vi "Weather Parse Test.vi"() -> ()   [LabVIEW 2020, in "CDM-Config.lvlib"] (continued)
\"NationalWeatherService\": [\n                        \"SCY\"\n                    ]\n                }\n            }\n        },\n        {\n            \"id\": \"https://api.weather.gov/alerts/urn:oid:2.49.0.1.840.0.85cfcb06bd0c86092fff4359af75aac0fabec681.004.1\",\n            \"type\": \"Feature\",\n            \"geometry\": null,\n            \"properties\": {\n                \"@id\": \"https://api.weather.gov/alerts/urn:oid:2.49.0.1.840.0.85cfcb06bd0c86092fff4359af75aac0fabec681.004.1\",\n                \"@type\": \"wx:Alert\",\n                \"id\": \"urn:oid:2.49.0.1.840.0.85cfcb06bd0c86092fff4359af75aac0fabec681.004.1\",\n                \"areaDesc\": \"Coastal waters from Cape Mendocino to Pt. Arena CA out 10 nm\",\n                \"geocode\": {\n                    \"SAME\": [\n                        \"057455\"\n                    ],\n                    \"UGC\": [\n                        \"PZZ455\"\n                    ]\n                },\n                \"affectedZones\": [\n                    \"https://api.weather.gov/zones/forecast/PZZ455\"\n                ],\n                \"references\": [\n                    {\n                        \"@id\": \"https://api.weather.gov/alerts/urn:oid:2.49.0.1.840.0.60f47e7d527764f0ce222d0fcb908b2519fae517.003.1\",\n                        \"identifier\": \"urn:oid:2.49.0.1.840.0.60f47e7d527764f0ce222d0fcb908b2519fae517.003.1\",\n                        \"sender\": \"w-nws.webmaster@noaa.gov\",\n                        \"sent\": \"2025-12-03T03:17:00-08:00\"\n                    }\n                ],\n                \"sent\": \"2025-12-03T07:39:00-08:00\",\n                \"effective\": \"2025-12-03T07:39:00-08:00\",\n                \"onset\": \"2025-12-03T07:39:00-08:00\",\n                \"expires\": \"2025-12-03T10:00:00-08:00\",\n                \"ends\": \"2025-12-03T10:00:00-08:00\",\n                \"status\": \"Actual\",\n                \"messageType\": \"Update\",\n                \"category\": \"Met\",\n                \"severity\": \"Minor\",\n                \"certainty\": \"Likely\",\n                \"urgency\": \"Expected\",\n                \"event\": \"Small Craft Advisory\",\n                \"sender\": \"w-nws.webmaster@noaa.gov\",\n                \"senderName\": \"NWS Eureka CA\",\n                \"headline\": \"Small Craft Advisory issued December 3 at 7:39AM PST until December 3 at 10:00AM PST by NWS Eureka CA\",\n                \"description\": \"* WHAT...North winds 10 to 20 kt with gusts up to 25 kt and seas\\n8 to 10 feet.\\n\\n* WHERE...Cape Mendocino to Pt Arena out 10 nm.\\n\\n* WHEN...Until 10 AM PST this morning.\\n\\n* IMPACTS...Conditions will be hazardous to small craft.\",\n                \"instruction\": \"Inexperienced mariners, especially those operating smaller\\nvessels, should avoid navigating in hazardous conditions.\",\n                \"response\": \"Avoid\",\n                \"parameters\": {\n                    \"AWIPSidentifier\": [\n                        \"MWWEKA\"\n                    ],\n                    \"WMOidentifier\": [\n                        \"WHUS76 KEKA 031539\"\n                    ],\n                    \"NWSheadline\": [\n                        \"SMALL CRAFT ADVISORY REMAINS IN EFFECT UNTIL 10 AM PST THIS MORNING\"\n                    ],\n                    \"BLOCKCHANNEL\": [\n                        \"EAS\",\n                        \"NWEM\",\n                        \"CMAS\"\n                    ],\n                    \"VTEC\": [\n                        \"/O.CON.KEKA.SC.Y.0131.000000T0000Z-251203T1800Z/\"\n                    ],\n                    \"eventEndingTime\": [\n                        \"2025-12-03T10:00:00-08:00\"\n                    ],\n                    \"expiredReferences\": [\n                        \"w-nws.webmaster@noaa.gov,urn:oid:2.49.0.1.840.0.abe195d0561fd25b031b5bfec9df0b944a5ace40.003.1,2025-12-02T21:50:00-08:00 w-nws.webmaster@noaa.gov,urn:oid:2.49.0.1.840.0.e32ecb5cf39de3c0d1e2da73c56319d7880d5ad3.004.1,2025-12-02T15:45:00-08:00 w-nws.webmaster@noaa.gov,urn:oid:2.49.0.1.840.0.e0b91c1e8c9c801e386b75444bbd2a0bbc5299eb.004.1,2025-12-02T14:39:00-08:00 w-nws.webmaster@noaa.gov,urn:oid:2.49.0.1.840.0.0a5dc3462cdc1726ad314e876783ee5bf7071762.004.1,2025-12-02T09:55:00-08:00 w-nws.webmaster@noaa.gov,urn:oid:2.49.0.1.840.0.01de2552a96f0b556f81f7a24cea9bae9b7d39b8.003.1,2025-12-02T03:48:00-08:00 w-nws.webmaster@noaa.gov,urn:oid:2.49.0.1.840.0.ca2f9b9bc4efc4c7ec6c14c74d7b35cc28fee802.003.1,2025-12-01T20:59:00-08:00 w-nws.webmaster@noaa.gov,urn:oid:2.49.0.1.840.0.341d2d3541a24810a337eb1f7ebd4af858289c9a.003.1,2025-12-01T14:59:00-08:00 w-nws.webmaster@noaa.gov,urn:oid:2.49.0.1.840.0.e0da5ffb117eb3eb07d4855bb3809c65d8bd08ee.001.1,2025-11-30T22:46:00-08:00 w-nws.webmaster@noaa.gov,urn:oid:2.49.0.1.840.0.3141b440711a7dab2caf67b4d892f368eedce3a1.001.1,2025-11-30T15:10:00-08:00 w-nws.webmaster@noaa.gov,urn:oid:2.49.0.1.840.0.61c600a3fee31e0c5b3344407f02fbb11b4030f7.003.1,2025-11-30T11:25:00-08:00 w-nws.webmaster@noaa.gov,urn:oid:2.49.0.1.840.0.475fbd03966c809e753c380c88b8f5a7913fc370.001.1,2025-11-30T02:23:00-08:00 w-nws.webmaster@noaa.gov,urn:oid:2.49.0.1.840.0.456ac22e39df6d72b640469b5ee3cd6819367cee.001.1,2025-11-29T22:41:00-08:00 w-nws.webmaster@noaa.gov,urn:oid:2.49.0.1.840.0.3f2569b420bbe6dab1f5676473753e2d387027f5.001.1,2025-11-29T15:01:00-08:00 w-nws.webmaster@noaa.gov,urn:oid:2.49.0.1.840.0.558b96257a3d492dbe31195be5d89212c36df85e.003.1,2025-11-29T10:51:00-08:00 w-nws.webmaster@noaa.gov,urn:oid:2.49.0.1.840.0.96be26edb9a6c9dcbf7df831b0453d5650027364.001.1,2025-11-29T02:25:00-08:00 w-nws.webmaster@noaa.gov,urn:oid:2.49.0.1.840.0.c3b1f937b5abbc5ea56d2724b02e758aa1c01179.002.1,2025-11-28T22:31:00-08:00 w-nws.webmaster@noaa.gov,urn:oid:2.49.0.1.840.0.e3db8e512cec14c9022bfe9f2c10ba787d2e6b8d.001.1,2025-11-28T11:48:00-08:00\"\n                    ]\n                },\n                \"scope\": \"Public\",\n                \"code\": \"IPAWSv1.0\",\n                \"language\": \"en-US\",\n                \"web\": \"http://www.weather.gov\",\n                \"eventCode\": {\n                    \"SAME\": [\n                        \"NWS\"\n                    ],\n                    \"NationalWeatherService\": [\n                        \"SCY\"\n                    ]\n                }\n            }\n        },\n        {\n            \"id\": \"https://api.weather.gov/alerts/urn:oid:2.49.0.1.840.0.220f0a3be3b6cd2f2d64124491430aaf409f9b6f.001.1\",\n            \"type\": \"Feature\",\n            \"geometry\": null,\n            \"properties\": {\n                \"@id\": \"https://api.weather.gov/alerts/urn:oid:2.49.0.1.840.0.220f0a3be3b6cd2f2d64124491430aaf409f9b6f.001.1\",\n                \"@type\": \"wx:Alert\",\n                \"id\": \"urn:oid:2.49.0.1.840.0.220f0a3be3b6cd2f2d64124491430aaf409f9b6f.001.1\",\n                \"areaDesc\": \"Western Chippewa; Central Chippewa\",\n                \"geocode\": {\n                    \"SAME\": [\n                        \"026033\"\n                    ],\n                    \"UGC\": [\n                        \"MIZ086\",\n                        \"MIZ087\"\n                    ]\n                },\n                \"affectedZones\": [\n                    \"https://api.weather.gov/zones/forecast/MIZ086\",\n                    \"https://api.weather.gov/zones/forecast/MIZ087\"\n                ],\n                \"references\": [\n                    {\n                        \"@id\": \"https://api.weather.gov/alerts/urn:oid:2.49.0.1.840.0.68f3b48d66caf3405fc5bfbb1a371148b61f2b0f.001.1\",\n                        \"identifier\": \"urn:oid:2.49.0.1.840.0.68f3b48d66caf3405fc5bfbb1a371148b61f2b0f.001.1\",\n                        \"sender\": \"w-nws.webmaster@noaa.gov\",\n                        \"sent\": \"2025-12-03T02:53:00-05:00\"\n                    }\n                ],\n                \"sent\": \"2025-12-03T10:36:00-05:00\",\n                \"effective\": \"2025-12-03T10:36:00-05:00\",\n                \"onset\": \"2025-12-03T13:00:00-05:00\",\n                \"expires\": \"2025-12-03T22:45:00-05:00\",\n                \"ends\": \"2025-12-04T13:00:00-05:00\",\n                \"status\": \"Actual\",\n                \"messageType\": \"Update\",\n                \"category\": \"Met\",\n                \"severity\": \"Severe\",\n                \"certainty\": \"Likely\",\n                \"urgency\": \"Expected\",\n                \"event\": \"Winter Storm Warning\",\n                \"sender\": \"w-nws.webmaster@noaa.gov\",\n                \"senderName\": \"NWS Gaylord MI\",\n                \"headline\": \"Winter Storm Warning issued December 3 at 10:36AM EST until December 4 at 1:00PM EST by NWS Gaylord MI\",\n                \"description\": \"* WHAT...Heavy snow expected. Total snow accumulations between 6 and\\n12 inches, locally higher amounts possible. Winds gusting between\\n25 and 30 mph will result in blowing snow at times.\\n\\n* WHERE...Central Chippewa and Western Chippewa Counties.\\n\\n* WHEN...Until 1 PM EST Thursday.\\n\\n* IMPACTS...Visibilities may drop below 1/4 mile due to falling and\\nblowing snow. Travel could be very difficult. The hazardous\\nconditions will impact the Thursday morning commute.\",\n                \"instruction\": \"If you must travel, keep an extra flashlight, food, and water in\\nyour vehicle in case of an emergency.\\n\\nIf travel is absolutely necessary, drive with extreme caution and be\\nprepared for sudden changes in visibility. Leave plenty of room\\nbetween you and the motorist ahead of you, and allow extra time to\\nreach your destination. Avoid sudden braking or acceleration, and be\\nespecially cautious on hills or when making turns. Make sure your\\ncar is winterized and in good working order.\",\n                \"response\": \"Prepare\",\n                \"parameters\": {\n                    \"AWIPSidentifier\": [\n                        \"WSWAPX\"\n                    ],\n                    \"WMOidentifier\": [\n                        \"WWUS43 KAPX 031536\"\n                    ],\n                    \"NWSheadline\": [\n                        \"WINTER STORM WARNING REMAINS IN EFFECT UNTIL 1 PM EST THURSDAY\"\n                    ],\n                    \"BLOCKCHANNEL\": [\n                        \"EAS\",\n                        \"NWEM\",\n                        \"CMAS\"\n                    ],\n                    \"EAS-ORG\": [\n                        \"WXR\"\n                    ],\n                    \"VTEC\": [\n                        \"/O.CON.KAPX.WS.W.0014.251203T1800Z-251204T1800Z/\"\n                    ],\n                    \"eventEndingTime\": [\n                        \"2025-12-04T13:00:00-05:00\"\n                    ]\n                },\n                \"scope\": \"Public\",\n                \"code\": \"IPAWSv1.0\",\n                \"language\": \"en-US\",\n                \"web\": \"http://www.weather.gov\",\n                \"eventCode\": {\n                    \"SAME\": [\n                        \"WSW\"\n                    ],\n                    \"NationalWeatherService\": [\n                        \"WSW\"\n                    ]\n                }\n            }\n        },\n        {\n            \"id\": \"https://api.weather.gov/alerts/urn:oid:2.49.0.1.840.0.70532f7794760aa59fb14677883cbb330aad0f90.001.1\",\n            \"type\": \"Feature\",\n            \"geometry\": null,\n            \"properties\": {\n                \"@id\": \"https://api.weather.gov/alerts/urn:oid:2.49.0.1.840.0.70532f7794760aa59fb14677883cbb330aad0f90.001.1\",\n                \"@type\": \"wx:Alert\",\n                \"id\": \"urn:oid:2.49.0.1.840.0.70532f7794760aa59fb14677883cbb330aad0f90.001.1\",\n                \"areaDesc\": \"New Buffalo MI to St Joseph MI; Michigan City IN to New Buffalo MI\",\n                \"geocode\": {\n                    \"SAME\": [\n                        \"092043\",\n                        \"092046\"\n                    ],\n                    \"UGC\": [\n                        \"LMZ043\",\n                        \"LMZ046\"\n                    ]\n                },\n                \"affectedZones\": [\n                    \"https://api.weather.gov/zones/forecast/LMZ043\",\n                    \"https://api.weather.gov/zones/forecast/LMZ046\"\n                ],\n                \"references\": [\n                    {\n                        \"@id\": \"https://api.weather.gov/alerts/urn:oid:2.49.0.1.840.0.875506e3e040bbcc4b2fc71b1eece95556c3b51a.001.1\",\n                        \"identifier\": \"urn:oid:2.49.0.1.840.0.875506e3e040bbcc4b2fc71b1eece95556c3b51a.001.1\",\n                        \"sender\": \"w-nws.webmaster@noaa.gov\",\n                        \"sent\": \"2025-12-03T04:19:00-05:00\"\n                    }\n                ],\n                \"sent\": \"2025-12-03T10:28:00-05:00\",\n                \"effective\": \"2025-12-03T10:28:00-05:00\",\n                \"onset\": \"2025-12-03T10:28:00-05:00\",\n                \"expires\": \"2025-12-03T18:30:00-05:00\",\n                \"ends\": \"2025-12-04T19:00:00-05:00\",\n                \"status\": \"Actual\",\n                \"messageType\": \"Update\",\n                \"category\": \"Met\",\n                \"severity\": \"Minor\",\n                \"certainty\": \"Likely\",\n                \"urgency\": \"Expected\",\n                \"event\": \"Small Craft Advisory\",\n                \"sender\": \"w-nws.webmaster@noaa.gov\",\n                \"senderName\": \"NWS Northern Indiana\",\n                \"headline\": \"Small Craft Advisory issued December 3 at 10:28AM EST until December 4 at 7:00PM EST by NWS Northern Indiana\",\n                \"description\": \"* WHAT...Southwest 15 to 25 knots becoming northwest with gusts\\nup to 25 to 30 knots and waves 6 to 9 feet.\\n\\n* WHERE...Michigan City IN to St Joseph MI.\\n\\n* WHEN...Until 7 PM EST Thursday.\\n\\n* IMPACTS...Conditions will be hazardous to small craft.\",\n                \"instruction\": \"Inexperienced mariners, especially those operating smaller\\nvessels, should avoid navigating in hazardous conditions.\",\n                \"response\": \"Avoid\",\n                \"parameters\": {\n                    \"AWIPSidentifier\": [\n                        \"MWWIWX\"\n                    ],\n                    \"WMOidentifier\": [\n                        \"WHUS73 KIWX 031528\"\n                    ],\n                    \"NWSheadline\": [\n                        \"SMALL CRAFT ADVISORY REMAINS IN EFFECT UNTIL 7 PM EST THURSDAY\"\n                    ],\n                    \"BLOCKCHANNEL\": [\n                        \"EAS\",\n                        \"NWEM\",\n                        \"CMAS\"\n                    ],\n                    \"VTEC\": [\n                        \"/O.CON.KIWX.SC.Y.0073.000000T0000Z-251205T0000Z/\"\n                    ],\n                    \"eventEndingTime\": [\n                        \"2025-12-04T19:00:00-05:00\"\n                    ],\n                    \"expiredReferences\": [\n                        \"w-nws.webmaster@noaa.gov,urn:oid:2.49.0.1.840.0.225142cd75165574bdad700dfb60a5d5354b40a4.001.1,2025-12-02T21:13:00-05:00 w-nws.webmaster@noaa.gov,urn:oid:2.49.0.1.840.0.a0e704ec5a442f14cfca1d10613311a0e02b15c6.001.1,2025-12-02T15:47:00-05:00 w-nws.webmaster@noaa.gov,urn:oid:2.49.0.1.840.0.6b2791b857a86681ce998af8adb83a08b01f25a5.001.1,2025-12-02T11:04:00-05:00 w-nws.webmaster@noaa.gov,urn:oid:2.49.0.1.840.0.a57567c3b2042ce4a02e8b09eda0f6c7e7ccc8d7.001.1,2025-12-02T03:51:00-05:00\"\n                    ]\n                },\n                \"scope\": \"Public\",\n                \"code\": \"IPAWSv1.0\",\n                \"language\": \"en-US\",\n                \"web\": \"http://www.weather.gov\",\n                \"eventCode\": {\n                    \"SAME\": [\n                        \"NWS\"\n                    ],\n                    \"NationalWeatherService\": [\n                        \"SCY\"\n                    ]\n                }\n            }\n        },\n        {\n            \"id\": \"https://api.weather.gov/alerts/urn:oid:2.49.0.1.840.0.296069c17a90f6e5215450afb7029362483104e1.002.1\",\n            \"type\": \"Feature\",\n            \"geometry\": null,\n            \"properties\": {\n                \"@id\": \"https://api.weather.gov/alerts/urn:oid:2.49.0.1.840.0.296069c17a90f6e5215450afb7029362483104e1.002.1\",\n                \"@type\": \"wx:Alert\",\n                \"id\": \"urn:oid:2.49.0.1.840.0.296069c17a90f6e5215450afb7029362483104e1.002.1\",\n                \"areaDesc\": \"Northern Sangre de Cristo Mountains Between 8500 And 11000 Ft; Northern Sangre de Cristo Mountains above 11000 Ft; Southern Sangre De Cristo Mountains Between 7500 and 11000 Ft; Southern Sangre De Cristo Mountains Above 11000 Ft\",\n                \"geocode\": {\n                    \"SAME\": [\n                        \"008003\",\n                        \"008015\",\n                        \"008023\",\n                        \"008027\",\n                        \"008043\",\n                        \"008055\",\n                        \"008109\",\n                        \"008071\"\n                    ],\n                    \"UGC\": [\n                        \"COZ072\",\n                        \"COZ073\",\n                        \"COZ074\",\n                        \"COZ075\"\n                    ]\n                },\n                \"affectedZones\": [\n                    \"https://api.weather.gov/zones/forecast/COZ072\",\n                    \"https://api.weather.gov/zones/forecast/COZ073\",\n                    \"https://api.weather.gov/zones/forecast/COZ074\",\n                    \"https://api.weather.gov/zones/forecast/COZ075\"\n                ],\n                \"references\": [\n                    {\n                        \"@id\": \"https://api.weather.gov/alerts/urn:oid:2.49.0.1.840.0.f1520a771888f2286c7e9f041b0899cca2ffbe10.001.1\",\n                        \"identifier\": \"urn:oid:2.49.0.1.840.0.f1520a771888f2286c7e9f041b0899cca2ffbe10.001.1\",\n                        \"sender\": \"w-nws.webmaster@noaa.gov\",\n                        \"sent\": \"2025-12-03T00:40:00-07:00\"\n                    },\n                    {\n                        \"@id\": \"https://api.weather.gov/alerts/urn:oid:2.49.0.1.840.0.3e97ab4a6a3c23a3a20405d82b018ef9927db31d.002.1\",\n                        \"identifier\": \"urn:oid:2.49.0.1.840.0.3e97ab4a6a3c23a3a20405d82b018ef9927db31d.002.1\",\n                        \"sender\": \"w-nws.webmaster@noaa.gov\",\n                        \"sent\": \"2025-12-03T00:46:00-07:00\"\n                    },\n                    {\n                        \"@id\": \"https://api.weather.gov/alerts/urn:oid:2.49.0.1.840.0.b7b2384d0cd65fff536137c85933eace889e9254.001.1\",\n                        \"identifier\": \"urn:oid:2.49.0.1.840.0.b7b2384d0cd65fff536137c85933eace889e9254.001.1\",\n                        \"sender\": \"w-nws.webmaster@noaa.gov\",\n                        \"sent\": \"2025-12-03T00:53:00-07:00\"\n                    },\n                    {\n                        \"@id\": \"https://api.weather.gov/alerts/urn:oid:2.49.0.1.840.0.5bb2b589973a618ffa88ed552c21d1806fce1897.001.1\",\n                        \"identifier\": \"urn:oid:2.49.0.1.840.0.5bb2b589973a618ffa88ed552c21d1806fce1897.001.1\",\n                        \"sender\": \"w-nws.webmaster@noaa.gov\",\n                        \"sent\": \"2025-12-03T02:10:00-07:00\"\n                    }\n                ],\n                \"sent\": \"2025-12-03T08:17:00-07:00\",\n                \"effective\": \"2025-12-03T08:17:00-07:00\",\n                \"onset\": \"2025-12-03T08:17:00-07:00\",\n                \"expires\": \"2025-12-03T16:30:00-07:00\",\n                \"ends\": \"2025-12-04T02:00:00-07:00\",\n                \"status\": \"Actual\",\n                \"messageType\": \"Update\",\n                \"category\": \"Met\",\n                \"severity\": \"Severe\",\n                \"certainty\": \"Likely\",\n                \"urgency\": \"Expected\",\n                \"event\": \"Winter Storm Warning\",\n                \"sender\": \"w-nws.webmaster@noaa.gov\",\n                \"senderName\": \"NWS Pueblo CO\",\n                \"headline\": \"Winter Storm Warning issued December 3 at 8:17AM MST until December 4 at 2:00AM MST by NWS Pueblo CO\",\n                \"description\": \"* WHAT...Heavy snow expected. Total snow accumulations between 8 to\\n20 inches.\\n\\n* WHERE...Sangre de Cristo Mountains.\\n\\n* WHEN...Until 2 AM MST Thursday.\\n\\n* IMPACTS...Travel could be very difficult to impossible. The\\nhazardous conditions could impact the Wednesday evening commute.\",\n                \"instruction\": \"If you must travel, keep an extra flashlight, food, and water in\\nyour vehicle in case of an emergency. The latest road conditions for\\nthe state you are calling from can be obtained by calling 5 1 1.\\n\\nPersons should consider delaying all travel. Motorists should use\\nextreme caution if travel is absolutely necessary.\",\n                \"response\": \"Prepare\",\n                \"parameters\": {\n                    \"AWIPSidentifier\": [\n                        \"WSWPUB\"\n                    ],\n                    \"WMOidentifier\": [\n                        \"WWUS45 KPUB 031517\"\n                    ],\n                    \"NWSheadline\": [\n                        \"WINTER STORM WARNING REMAINS IN EFFECT UNTIL 2 AM MST THURSDAY\"\n                    ],\n                    \"BLOCKCHANNEL\": [\n                        \"EAS\",\n                        \"NWEM\",\n                        \"CMAS\"\n                    ],\n                    \"EAS-ORG\": [\n                        \"WXR\"\n                    ],\n                    \"VTEC\": [\n                        \"/O.CON.KPUB.WS.W.0011.000000T0000Z-251204T0900Z/\"\n                    ],\n                    \"eventEndingTime\": [\n                        \"2025-12-04T02:00:00-07:00\"\n                    ],\n                    \"expiredReferences\": [\n                        \"w-nws.webmaster@noaa.gov,urn:oid:2.49.0.1.840.0.1683fac8dbbcced155b8c3ee102b504a61d03b48.001.1,2025-12-02T21:22:00-07:00 w-nws.webmaster@noaa.gov,urn:oid:2.49.0.1.840.0.3af7c19979dcb0fd957b60f169e1bc971c265b37.001.2,2025-12-02T14:07:00-07:00\"\n                    ]\n                },\n                \"scope\": \"Public\",\n                \"code\": \"IPAWSv1.0\",\n                \"language\": \"en-US\",\n                \"web\": \"http://www.weather.gov\",\n                \"eventCode\": {\n                    \"SAME\": [\n                        \"WSW\"\n                    ],\n                    \"NationalWeatherService\": [\n                        \"WSW\"\n                    ]\n                }\n            }\n        },\n        {\n            \"id\": \"https://api.weather.gov/alerts/urn:oid:2.49.0.1.840.0.296069c17a90f6e5215450afb7029362483104e1.001.2\",\n            \"type\": \"Feature\",\n            \"geometry\": null,\n            \"properties\": {\n                \"@id\": \"https://api.weather.gov/alerts/urn:oid:2.49.0.1.840.0.296069c17a90f6e5215450afb7029362483104e1.001.2\",\n                \"@type\": \"wx:Alert\",\n                \"id\": \"urn:oid:2.49.0.1.840.0.296069c17a90f6e5215450afb7029362483104e1.001.2\",\n                \"areaDesc\": \"Wet Mountain Valley Below 8500 Ft; Wet Mountains between 6300 and 10000Ft; Wet Mountains above 10000 Ft; Walsenburg Vicinity/Upper Huerfano River Basin Below 7500 Ft\",\n                \"geocode\": {\n                    \"SAME\": [\n                        \"008027\",\n                        \"008055\",\n                        \"008043\",\n                        \"008101\"\n                    ],\n                    \"UGC\": [\n                        \"COZ078\",\n                        \"COZ079\",\n                        \"COZ080\",\n                        \"COZ087\"\n                    ]\n                },\n                \"affectedZones\": [\n                    \"https://api.weather.gov/zones/forecast/COZ078\",\n                    \"https://api.weather.gov/zones/forecast/COZ079\",\n                    \"https://api.weather.gov/zones/forecast/COZ080\",\n                    \"https://api.weather.gov/zones/forecast/COZ087\"\n                ],\n                \"references\": [],\n                \"sent\": \"2025-12-03T08:17:00-07:00\",\n                \"effective\": \"2025-12-03T08:17:00-07:00\",\n                \"onset\": \"2025-12-03T08:17:00-07:00\",\n                \"expires\": \"2025-12-03T16:30:00-07:00\",\n                \"ends\": \"2025-12-04T02:00:00-07:00\",\n                \"status\": \"Actual\",\n                \"messageType\": \"Alert\",\n                \"category\": \"Met\",\n                \"severity\": \"Severe\",\n                \"certainty\": \"Likely\",\n                \"urgency\": \"Expected\",\n                \"event\": \"Winter Storm Warning\",\n                \"sender\": \"w-nws.webmaster@noaa.gov\",\n                \"senderName\": \"NWS Pueblo CO\",\n                \"headline\": \"Winter Storm Warning issued December 3 at 8:17AM MST until December 4 at 2:00AM MST by NWS Pueblo CO\",\n                \"description\": \"* WHAT...Heavy snow. Additional snow accumulations between 8 and 16\\ninches. The heaviest amounts are expected along the eastern slopes\\nof the Wet Mountains.\\n\\n* WHERE...Wet Mountains, Wet Mountain Valley, and Walsenburg\\nVicinity/Upper Huerfano River Basin Below 7500 Feet.\\n\\n* WHEN...Until 2 AM MST Thursday.\\n\\n* IMPACTS...Travel could be very difficult to impossible. The\\nhazardous conditions could impact the Wednesday evening commute.\",\n                \"instruction\": \"If you must travel, keep an extra flashlight, food, and water in\\nyour vehicle in case of an emergency. The latest road conditions for\\nthe state you are calling from can be obtained by calling 5 1 1.\\n\\nPersons should consider delaying all travel. Motorists should use\\nextreme caution if travel is absolutely necessary.\",\n                \"response\": \"Prepare\",\n                \"parameters\": {\n                    \"AWIPSidentifier\": [\n                        \"WSWPUB\"\n                    ],\n                    \"WMOidentifier\": [\n                        \"WWUS45 KPUB 031517\"\n                    ],\n                    \"NWSheadline\": [\n                        \"WINTER STORM WARNING IN EFFECT UNTIL 2 AM MST THURSDAY\"\n                    ],\n                    \"BLOCKCHANNEL\": [\n                        \"EAS\",\n                        \"NWEM\",\n                        \"CMAS\"\n                    ],\n                    \"EAS-ORG\": [\n                        \"WXR\"\n                    ],\n                    \"VTEC\": [\n                        \"/O.EXA.KPUB.WS.W.0011.000000T0000Z-251204T0900Z/\"\n                    ],\n                    \"eventEndingTime\": [\n                        \"2025-12-04T02:00:00-07:00\"\n                    ]\n                },\n                \"scope\": \"Public\",\n                \"code\": \"IPAWSv1.0\",\n                \"language\": \"en-US\",\n                \"web\": \"http://www.weather.gov\",\n                \"eventCode\": {\n                    \"SAME\": [\n                        \"WSW\"\n                    ],\n                    \"NationalWeatherService\": [\n                        \"WSW\"\n                    ]\n                }\n            }\n        },\n        {\n            \"id\": \"https://api.weather.gov/alerts/urn:oid:2.49.0.1.840.0.296069c17a90f6e5215450afb7029362483104e1.008.1\",\n            \"type\": \"Feature\",\n            \"geometry\": null,\n            \"properties\": {\n                \"@id\": \"https://api.weather.gov/alerts/urn:oid:2.49.0.1.840.0.296069c17a90f6e5215450afb7029362483104e1.008.1\",\n                \"@type\": \"wx:Alert\",\n                \"id\": \"urn:oid:2.49.0.1.840.0.296069c17a90f6e5215450afb7029362483104e1.008.1\",\n                \"areaDesc\": \"Teller County/Rampart Range above 7500fT/Pike's Peak Between 7500 And 11000 Ft; Pikes Peak above 11000 Ft; Northern El Paso County/Monument Ridge/Rampart Range Below 7500 Ft\",\n                \"geocode\": {\n                    \"SAME\": [\n                        \"008041\",\n                        \"008043\",\n                        \"008119\"\n                    ],\n                    \"UGC\": [\n                        \"COZ081\",\n                        \"COZ082\",\n                        \"COZ084\"\n                    ]\n                },\n                \"affectedZones\": [\n                    \"https://api.weather.gov/zones/forecast/COZ081\",\n                    \"https://api.weather.gov/zones/forecast/COZ082\",\n                    \"https://api.weather.gov/zones/forecast/COZ084\"\n                ],\n                \"references\": [\n                    {\n                        \"@id\": \"https://api.weather.gov/alerts/urn:oid:2.49.0.1.840.0.f1520a771888f2286c7e9f041b0899cca2ffbe10.005.1\",\n                        \"identifier\": \"urn:oid:2.49.0.1.840.0.f1520a771888f2286c7e9f041b0899cca2ffbe10.005.1\",\n                        \"sender\": \"w-nws.webmaster@noaa.gov\",\n                        \"sent\": \"2025-12-03T00:40:00-07:00\"\n                    },\n                    {\n                        \"@id\": \"https://api.weather.gov/alerts/urn:oid:2.49.0.1.840.0.3e97ab4a6a3c23a3a20405d82b018ef9927db31d.005.1\",\n                        \"identifier\": \"urn:oid:2.49.0.1.840.0.3e97ab4a6a3c23a3a20405d82b018ef9927db31d.005.1\",\n                        \"sender\": \"w-nws.webmaster@noaa.gov\",\n                        \"sent\": \"2025-12-03T00:46:00-07:00\"\n                    },\n                    {\n                        \"@id\": \"https://api.weather.gov/alerts/urn:oid:2.49.0.1.840.0.b7b2384d0cd65fff536137c85933eace889e9254.005.1\",\n                        \"identifier\": \"urn:oid:2.49.0.1.840.0.b7b2384d0cd65fff536137c85933eace889e9254.005.1\",\n                        \"sender\": \"w-nws.webmaster@noaa.gov\",\n                        \"sent\": \"2025-12-03T00:53:00-07:00\"\n                    },\n                    {\n                        \"@id\": \"https://api.weather.gov/alerts/urn:oid:2.49.0.1.840.0.5bb2b589973a618ffa88ed552c21d1806fce1897.004.1\",\n                        \"identifier\": \"urn:oid:2.49.0.1.840.0.5bb2b589973a618ffa88ed552c21d1806fce1897.004.1\",\n                        \"sender\": \"w-nws.webmaster@noaa.gov\",\n                        \"sent\": \"2025-12-03T02:10:00-07:00\"\n                    }\n                ],\n                \"sent\": \"2025-12-03T08:17:00-07:00\",\n                \"effective\": \"2025-12-03T08:17:00-07:00\",\n                \"onset\": \"2025-12-03T08:17:00-07:00\",\n                \"expires\": \"2025-12-03T16:30:00-07:00\",\n                \"ends\": \"2025-12-03T20:00:00-07:00\",\n                \"status\": \"Actual\",\n                \"messageType\": \"Update\",\n                \"category\": \"Met\",\n                \"severity\": \"Moderate\",\n                \"certainty\": \"Likely\",\n                \"urgency\": \"Expected\",\n                \"event\": \"Winter Weather Advisory\",\n                \"sender\": \"w-nws.webmaster@noaa.gov\",\n                \"senderName\": \"NWS Pueblo CO\",\n                \"headline\": \"Winter Weather Advisory issued December 3 at 8:17AM MST until December 3 at 8:00PM MST by NWS Pueblo CO\",\n                \"description\": \"* WHAT...Snow. Additional snow accumulations between 3 and 9 inches.\\nThe heaviest snow will fall this morning into early afternoon.\\n\\n* WHERE...Teller County and the Rampart Range including Pikes Peak,\\nand Northern El Paso.\\n\\n* WHEN...Until 8 PM MST this evening.\\n\\n* IMPACTS...Roads, and especially bridges and overpasses, will\\nlikely become slick and hazardous. Travel could be very difficult.\\nThe hazardous conditions could impact the Wednesday evening\\ncommute.\",\n                \"instruction\": \"Slow down and use caution while traveling. The latest road\\nconditions for the state you are calling from can be obtained by\\ncalling 5 1 1.\\n\\nBe prepared for slippery roads. Slow down and use caution while\\ndriving. If you are going outside, watch your first few steps taken\\non stairs, sidewalks, and driveways. These surfaces could be icy and\\nslippery, increasing your risk of a fall and injury.\",\n                \"response\": \"Execute\",\n                \"parameters\": {\n                    \"AWIPSidentifier\": [\n                        \"WSWPUB\"\n                    ],\n                    \"WMOidentifier\": [\n                        \"WWUS45 KPUB 031517\"\n                    ],\n                    \"NWSheadline\": [\n                        \"WINTER WEATHER ADVISORY REMAINS IN EFFECT UNTIL 8 PM MST THIS EVENING\"\n                    ],\n                    \"BLOCKCHANNEL\": [\n                        \"EAS\",\n                        \"NWEM\",\n                        \"CMAS\"\n                    ],\n                    \"VTEC\": [\n                        \"/O.CON.KPUB.WW.Y.0026.000000T0000Z-251204T0300Z/\"\n                    ],\n                    \"eventEndingTime\": [\n                        \"2025-12-03T20:00:00-07:00\"\n                    ],\n                    \"expiredReferences\": [\n                        \"w-nws.webmaster@noaa.gov,urn:oid:2.49.0.1.840.0.1683fac8dbbcced155b8c3ee102b504a61d03b48.004.1,2025-12-02T21:22:00-07:00 w-nws.webmaster@noaa.gov,urn:oid:2.49.0.1.840.0.3af7c19979dcb0fd957b60f169e1bc971c265b37.006.1,2025-12-02T14:07:00-07:00 w-nws.webmaster@noaa.gov,urn:oid:2.49.0.1.840.0.75fd3b8a9564f5fec4e84cc777455f52675d243c.001.1,2025-12-02T10:18:00-07:00 w-nws.webmaster@noaa.gov,urn:oid:2.49.0.1.840.0.db6c9ff9aeb621cf1cd0d104f439c64f55e7c3f7.001.1,2025-12-02T02:25:00-07:00\"\n                    ]\n                },\n                \"scope\": \"Public\",\n                \"code\": \"IPAWSv1.0\",\n                \"language\": \"en-US\",\n                \"web\": \"http://www.weather.gov\",\n                \"eventCode\": {\n                    \"SAME\": [\n                        \"NWS\"\n                    ],\n                    \"NationalWeatherService\": [\n                        \"WWY\"\n                    ]\n                }\n            }\n        },\n        {\n            \"id\": \"https://api.weather.gov/alerts/urn:oid:2.49.0.1.840.0.296069c17a90f6e5215450afb7029362483104e1.009.1\",\n            \"type\": \"Feature\",\n            \"geometry\": null,\n            \"properties\": {\n                \"@id\": \"https://api.weather.gov/alerts/urn:oid:2.49.0.1.840.0.296069c17a90f6e5215450afb7029362483104e1.009.1\",\n                \"@type\": \"wx:Alert\",\n                \"id\": \"urn:oid:2.49.0.1.840.0.296069c17a90f6e5215450afb7029362483104e1.009.1\",\n                \"areaDesc\": \"Trinidad Vicinity/Western Las Animas County Below 7500 Ft\",\n                \"geocode\": {\n                    \"SAME\": [\n                        \"008071\"\n                    ],\n                    \"UGC\": [\n                        \"COZ088\"\n                    ]\n                },\n                \"affectedZones\": [\n                    \"https://api.weather.gov/zones/forecast/COZ088\"\n                ],\n                \"references\": [\n                    {\n                        \"@id\": \"https://api.weather.gov/alerts/urn:oid:2.49.0.1.840.0.f1520a771888f2286c7e9f041b0899cca2ffbe10.008.1\",\n                        \"identifier\": \"urn:oid:2.49.0.1.840.0.f1520a771888f2286c7e9f041b0899cca2ffbe10.008.1\",\n                        \"sender\": \"w-nws.webmaster@noaa.gov\",\n                        \"sent\": \"2025-12-03T00:40:00-07:00\"\n                    },\n                    {\n                        \"@id\": \"https://api.weather.gov/alerts/urn:oid:2.49.0.1.840.0.3e97ab4a6a3c23a3a20405d82b018ef9927db31d.008.1\",\n                        \"identifier\": \"urn:oid:2.49.0.1.840.0.3e97ab4a6a3c23a3a20405d82b018ef9927db31d.008.1\",\n                        \"sender\": \"w-nws.webmaster@noaa.gov\",\n                        \"sent\": \"2025-12-03T00:46:00-07:00\"\n                    },\n                    {\n                        \"@id\": \"https://api.weather.gov/alerts/urn:oid:2.49.0.1.840.0.b7b2384d0cd65fff536137c85933eace889e9254.008.1\",\n                        \"identifier\": \"urn:oid:2.49.0.1.840.0.b7b2384d0cd65fff536137c85933eace889e9254.008.1\",\n                        \"sender\": \"w-nws.webmaster@noaa.gov\",\n                        \"sent\": \"2025-12-03T00:53:00-07:00\"\n                    },\n                    {\n                        \"@id\": \"https://api.weather.gov/alerts/urn:oid:2.49.0.1.840.0.5bb2b589973a618ffa88ed552c21d1806fce1897.008.1\",\n                        \"identifier\": \"urn:oid:2.49.0.1.840.0.5bb2b589973a618ffa88ed552c21d1806fce1897.008.1\",\n                        \"sender\": \"w-nws.webmaster@noaa.gov\",\n                        \"sent\": \"2025-12-03T02:10:00-07:00\"\n                    }\n                ],\n                \"sent\": \"2025-12-03T08:17:00-07:00\",\n                \"effective\": \"2025-12-03T08:17:00-07:00\",\n                \"onset\": \"2025-12-03T08:17:00-07:00\",\n                \"expires\": \"2025-12-03T16:30:00-07:00\",\n                \"ends\": \"2025-12-04T02:00:00-07:00\",\n                \"status\": \"Actual\",\n                \"messageType\": \"Update\",\n                \"category\": \"Met\",\n                \"severity\": \"Moderate\",\n                \"certainty\": \"Likely\",\n                \"urgency\": \"Expected\",\n                \"event\": \"Winter Weather Advisory\",\n                \"sender\": \"w-nws.webmaster@noaa.gov\",\n                \"senderName\": \"NWS Pueblo CO\",\n                \"headline\": \"Winter Weather Advisory issued December 3 at 8:17AM MST until December 4 at 2:00AM MST by NWS Pueblo CO\",\n                \"description\": \"* WHAT...Snow. Additional snow accumulations between 3 and 10 inches.\\n\\n* WHERE...Trinidad Vicinity/Western Las Animas County Below 7500\\nFeet.\\n\\n* WHEN...Until 2 AM MST Thursday.\\n\\n* IMPACTS...Roads, and especially bridges and overpasses, will\\nlikely become slick and hazardous. Travel could be very difficult.\\nThe hazardous conditions could impact the Wednesday evening\\ncommute.\",\n                \"instruction\": \"Slow down and use caution while traveling. The latest road\\nconditions for the state you are calling from can be obtained by\\ncalling 5 1 1.\\n\\nBe prepared for slippery roads. Slow down and use caution while\\ndriving. If you are going outside, watch your first few steps taken\\non stairs, sidewalks, and driveways. These surfaces could be icy and\\nslippery, increasing your risk of a fall and injury.\",\n                \"response\": \"Execute\",\n                \"parameters\": {\n                    \"AWIPSidentifier\": [\n                        \"WSWPUB\"\n                    ],\n                    \"WMOidentifier\": [\n                        \"WWUS45 KPUB 031517\"\n                    ],\n                    \"NWSheadline\": [\n                        \"WINTER WEATHER ADVISORY REMAINS IN EFFECT UNTIL 2 AM MST THURSDAY\"\n                    ],\n                    \"BLOCKCHANNEL\": [\n                        \"EAS\",\n                        \"NWEM\",\n                        \"CMAS\"\n                    ],\n                    \"VTEC\": [\n                        \"/O.CON.KPUB.WW.Y.0026.000000T0000Z-251204T0900Z/\"\n                    ],\n                    \"eventEndingTime\": [\n                        \"2025-12-04T02:00:00-07:00\"\n                    ],\n                    \"expiredReferences\": [\n                        \"w-nws.webmaster@noaa.gov,urn:oid:2.49.0.1.840.0.1683fac8dbbcced155b8c3ee102b504a61d03b48.007.1,2025-12-02T21:22:00-07:00 w-nws.webmaster@noaa.gov,urn:oid:2.49.0.1.840.0.3af7c19979dcb0fd957b60f169e1bc971c265b37.008.1,2025-12-02T14:07:00-07:00 w-nws.webmaster@noaa.gov,urn:oid:2.49.0.1.840.0.75fd3b8a9564f5fec4e84cc777455f52675d243c.002.1,2025-12-02T10:18:00-07:00 w-nws.webmaster@noaa.gov,urn:oid:2.49.0.1.840.0.db6c9ff9aeb621cf1cd0d104f439c64f55e7c3f7.002.1,2025-12-02T02:25:00-07:00\"\n                    ]\n                },\n                \"scope\": \"Public\",\n                \"code\": \"IPAWSv1.0\",\n                \"language\": \"en-US\",\n                \"web\": \"http://www.weather.gov\",\n                \"eventCode\": {\n                    \"SAME\": [\n                        \"NWS\"\n                    ],\n                    \"NationalWeatherService\": [\n                        \"WWY\"\n                    ]\n                }\n            }\n        },\n        {\n            \"id\": \"https://api.weather.gov/alerts/urn:oid:2.49.0.1.840.0.296069c17a90f6e5215450afb7029362483104e1.003.1\",\n            \"type\": \"Feature\",\n            \"geometry\": null,\n            \"properties\": {\n                \"@id\": \"https://api.weather.gov/alerts/urn:oid:2.49.0.1.840.0.296069c17a90f6e5215450afb7029362483104e1.003.1\",\n                \"@type\": \"wx:Alert\",\n                \"id\": \"urn:oid:2.49.0.1.840.0.296069c17a90f6e5215450afb7029362483104e1.003.1\",\n                \"areaDesc\": \"Eastern Sawatch Mountains above 11000 Ft; Western Chaffee County Between 9000 and 11000 Ft; Saguache County East of Continental Divide below 10000 Ft\",\n                \"geocode\": {\n                    \"SAME\": [\n                        \"008015\",\n                        \"008065\",\n                        \"008109\",\n                        \"008105\"\n                    ],\n                    \"UGC\": [\n                        \"COZ060\",\n                        \"COZ061\",\n                        \"COZ065\"\n                    ]\n                },\n                \"affectedZones\": [\n                    \"https://api.weather.gov/zones/forecast/COZ060\",\n                    \"https://api.weather.gov/zones/forecast/COZ061\",\n                    \"https://api.weather.gov/zones/forecast/COZ065\"\n                ],\n                \"references\": [\n                    {\n                        \"@id\": \"https://api.weather.gov/alerts/urn:oid:2.49.0.1.840.0.b7b2384d0cd65fff536137c85933eace889e9254.002.1\",\n                        \"identifier\": \"urn:oid:2.49.0.1.840.0.b7b2384d0cd65fff536137c85933eace889e9254.002.1\",\n                        \"sender\": \"w-nws.webmaster@noaa.gov\",\n                        \"sent\": \"2025-12-03T00:53:00-07:00\"\n                    },\n                    {\n                        \"@id\": \"https://api.weather.gov/alerts/urn:oid:2.49.0.1.840.0.5bb2b589973a618ffa88ed552c21d1806fce1897.005.1\",\n                        \"identifier\": \"urn:oid:2.49.0.1.840.0.5bb2b589973a618ffa88ed552c21d1806fce1897.005.1\",\n                        \"sender\": \"w-nws.webmaster@noaa.gov\",\n                        \"sent\": \"2025-12-03T02:10:00-07:00\"\n                    }\n                ],\n                \"sent\": \"2025-12-03T08:17:00-07:00\",\n                \"effective\": \"2025-12-03T08:17:00-07:00\",\n                \"onset\": \"2025-12-03T08:17:00-07:00\",\n                \"expires\": \"2025-12-03T16:30:00-07:00\",\n                \"ends\": \"2025-12-03T20:00:00-07:00\",\n                \"status\": \"Actual\",\n                \"messageType\": \"Update\",\n                \"category\": \"Met\",\n                \"severity\": \"Moderate\",\n                \"certainty\": \"Likely\",\n                \"urgency\": \"Expected\",\n                \"event\": \"Winter Weather Advisory\",\n                \"sender\": \"w-nws.webmaster@noaa.gov\",\n                \"senderName\": \"NWS Pueblo CO\",\n                \"headline\": \"Winter Weather Advisory issued December 3 at 8:17AM MST until December 3 at 8:00PM MST by NWS Pueblo CO\",\n                \"description\": \"* WHAT...Snow expected. Total snow accumulations between 5 and 8\\ninches. Most of the snow in the Sawatch range will fall south of\\nCottonwood Pass.\\n\\n* WHERE...Eastern Sawatch Mountains Above 11000 Feet, Saguache\\nCounty East of Continental Divide Below 10000 Feet, and Western\\nChaffee County Between 9000 and 11000 Feet.\\n\\n* WHEN...Until 8 PM MST this evening.\\n\\n* IMPACTS...Travel could be very difficult. The hazardous conditions\\ncould impact the Wednesday evening commute.\",\n                \"instruction\": \"Slow down and use caution while traveling. The latest road\\nconditions for the state you are calling from can be obtained by\\ncalling 5 1 1.\",\n                \"response\": \"Execute\",\n                \"parameters\": {\n                    \"AWIPSidentifier\": [\n                        \"WSWPUB\"\n                    ],\n                    \"WMOidentifier\": [\n                        \"WWUS45 KPUB 031517\"\n                    ],\n                    \"NWSheadline\": [\n                        \"WINTER WEATHER ADVISORY REMAINS IN EFFECT UNTIL 8 PM MST THIS EVENING\"\n                    ],\n                    \"BLOCKCHANNEL\": [\n                        \"EAS\",\n                        \"NWEM\",\n                        \"CMAS\"\n                    ],\n                    \"VTEC\": [\n                        \"/O.CON.KPUB.WW.Y.0026.000000T0000Z-251204T0300Z/\"\n                    ],\n                    \"eventEndingTime\": [\n                        \"2025-12-03T20:00:00-07:00\"\n                    ]\n                },\n                \"scope\": \"Public\",\n                \"code\": \"IPAWSv1.0\",\n                \"language\": \"en-US\",\n                \"web\": \"http://www.weather.gov\",\n                \"eventCode\": {\n                    \"SAME\": [\n                        \"NWS\"\n                    ],\n                    \"NationalWeatherService\": [\n                        \"WWY\"\n                    ]\n                }\n            }\n        },\n        {\n            \"id\": \"https://api.weather.gov/alerts/urn:oid:2.49.0.1.840.0.296069c17a90f6e5215450afb7029362483104e1.006.1\",\n            \"type\": \"Feature\",\n            \"geometry\": null,\n            \"properties\": {\n                \"@id\": \"https://api.weather.gov/alerts/urn:oid:2.49.0.1.840.0.296069c17a90f6e5215450afb7029362483104e1.006.1\",\n                \"@type\": \"wx:Alert\",\n                \"id\": \"urn:oid:2.49.0.1.840.0.296069c17a90f6e5215450afb7029362483104e1.006.1\",\n                \"areaDesc\": \"Del Norte Vicinity/Northern San Luis Valley Below 8500 Ft; Alamosa  Vicinity/Central San Luis Valley Below 8500 Ft; Southern San Luis Valley\",\n                \"geocode\": {\n                    \"SAME\": [\n                        \"008105\",\n                        \"008109\",\n                        \"008003\",\n                        \"008021\",\n                        \"008023\"\n                    ],\n                    \"UGC\": [\n                        \"COZ069\",\n                        \"COZ070\",\n                        \"COZ071\"\n                    ]\n                },\n                \"affectedZones\": [\n                    \"https://api.weather.gov/zones/forecast/COZ069\",\n                    \"https://api.weather.gov/zones/forecast/COZ070\",\n                    \"https://api.weather.gov/zones/forecast/COZ071\"\n                ],\n                \"references\": [\n                    {\n                        \"@id\": \"https://api.weather.gov/alerts/urn:oid:2.49.0.1.840.0.f1520a771888f2286c7e9f041b0899cca2ffbe10.007.1\",\n                        \"identifier\": \"urn:oid:2.49.0.1.840.0.f1520a771888f2286c7e9f041b0899cca2ffbe10.007.1\",\n                        \"sender\": \"w-nws.webmaster@noaa.gov\",\n                        \"sent\": \"2025-12-03T00:40:00-07:00\"\n                    },\n                    {\n                        \"@id\": \"https://api.weather.gov/alerts/urn:oid:2.49.0.1.840.0.3e97ab4a6a3c23a3a20405d82b018ef9927db31d.007.1\",\n                        \"identifier\": \"urn:oid:2.49.0.1.840.0.3e97ab4a6a3c23a3a20405d82b018ef9927db31d.007.1\",\n                        \"sender\": \"w-nws.webmaster@noaa.gov\",\n                        \"sent\": \"2025-12-03T00:46:00-07:00\"\n                    },\n                    {\n                        \"@id\": \"https://api.weather.gov/alerts/urn:oid:2.49.0.1.840.0.b7b2384d0cd65fff536137c85933eace889e9254.007.1\",\n                        \"identifier\": \"urn:oid:2.49.0.1.840.0.b7b2384d0cd65fff536137c85933eace889e9254.007.1\",\n                        \"sender\": \"w-nws.webmaster@noaa.gov\",\n                        \"sent\": \"2025-12-03T00:53:00-07:00\"\n                    },\n                    {\n                        \"@id\": \"https://api.weather.gov/alerts/urn:oid:2.49.0.1.840.0.5bb2b589973a618ffa88ed552c21d1806fce1897.007.1\",\n                        \"identifier\": \"urn:oid:2.49.0.1.840.0.5bb2b589973a618ffa88ed552c21d1806fce1897.007.1\",\n                        \"sender\": \"w-nws.webmaster@noaa.gov\",\n                        \"sent\": \"2025-12-03T02:10:00-07:00\"\n                    }\n                ],\n                \"sent\": \"2025-12-03T08:17:00-07:00\",\n                \"effective\": \"2025-12-03T08:17:00-07:00\",\n                \"onset\": \"2025-12-03T08:17:00-07:00\",\n                \"expires\": \"2025-12-03T16:30:00-07:00\",\n                \"ends\": \"2025-12-04T02:00:00-07:00\",\n                \"status\": \"Actual\",\n                \"messageType\": \"Update\",\n                \"category\": \"Met\",\n                \"severity\": \"Moderate\",\n                \"certainty\": \"Likely\",\n                \"urgency\": \"Expected\",\n                \"event\": \"Winter Weather Advisory\",\n                \"sender\": \"w-nws.webmaster@noaa.gov\",\n                \"senderName\": \"NWS Pueblo CO\",\n                \"headline\": \"Winter Weather Advisory issued December 3 at 8:17AM MST until December 4 at 2:00AM MST by NWS Pueblo CO\",\n                \"description\": \"* WHAT...Snow. Additional snow accumulations between 2 and 9 inches.\\n\\n* WHERE...San Luis Valley.\\n\\n* WHEN...Until 2 AM MST Thursday.\\n\\n* IMPACTS...Travel could be very difficult. The hazardous conditions\\ncould impact the Wednesday evening commute.\",\n                \"instruction\": \"Slow down and use caution while traveling. The latest road\\nconditions for the state you are calling from can be obtained by\\ncalling 5 1 1.\",\n                \"response\": \"Execute\",\n                \"parameters\": {\n                    \"AWIPSidentifier\": [\n                        \"WSWPUB\"\n                    ],\n                    \"WMOidentifier\": [\n                        \"WWUS45 KPUB 031517\"\n                    ],\n                    \"NWSheadline\": [\n                        \"WINTER WEATHER ADVISORY REMAINS IN EFFECT UNTIL 2 AM MST THURSDAY\"\n                    ],\n                    \"BLOCKCHANNEL\": [\n                        \"EAS\",\n                        \"NWEM\",\n                        \"CMAS\"\n                    ],\n                    \"VTEC\": [\n                        \"/O.CON.KPUB.WW.Y.0026.000000T0000Z-251204T0900Z/\"\n                    ],\n                    \"eventEndingTime\": [\n                        \"2025-12-04T02:00:00-07:00\"\n                    ],\n                    \"expiredReferences\": [\n                        \"w-nws.webmaster@noaa.gov,urn:oid:2.49.0.1.840.0.1683fac8dbbcced155b8c3ee102b504a61d03b48.006.1,2025-12-02T21:22:00-07:00 w-nws.webmaster@noaa.gov,urn:oid:2.49.0.1.840.0.3af7c19979dcb0fd957b60f169e1bc971c265b37.005.1,2025-12-02T14:07:00-07:00\"\n                    ]\n                },\n                \"scope\": \"Public\",\n                \"code\": \"IPAWSv1.0\",\n                \"language\": \"en-US\",\n                \"web\": \"http://www.weather.gov\",\n                \"eventCode\": {\n                    \"SAME\": [\n                        \"NWS\"\n                    ],\n                    \"NationalWeatherService\": [\n                        \"WWY\"\n                    ]\n                }\n            }\n        },\n        {\n            \"id\": \"https://api.weather.gov/alerts/urn:oid:2.49.0.1.840.0.296069c17a90f6e5215450afb7029362483104e1.005.1\",\n            \"type\": \"Feature\",\n            \"geometry\": null,\n            \"properties\": {\n                \"@id\": \"https://api.weather.gov/alerts/urn:oid:2.49.0.1.840.0.296069c17a90f6e5215450afb7029362483104e1.005.1\",\n                \"@type\": \"wx:Alert\",\n                \"id\": \"urn:oid:2.49.0.1.840.0.296069c17a90f6e5215450afb7029362483104e1.005.1\",\n                \"areaDesc\": \"La Garita Mountains Above 10000 Ft; Upper Rio Grande Valley/Eastern San Juan Mountains Below 10000 Ft; Eastern San Juan Mountains Above 10000 Ft\",\n                \"geocode\": {\n                    \"SAME\": [\n                        \"008079\",\n                        \"008105\",\n                        \"008109\",\n                        \"008021\"\n                    ],\n                    \"UGC\": [\n                        \"COZ066\",\n                        \"COZ067\",\n                        \"COZ068\"\n                    ]\n                },\n                \"affectedZones\": [\n                    \"https://api.weather.gov/zones/forecast/COZ066\",\n                    \"https://api.weather.gov/zones/forecast/COZ067\",\n                    \"https://api.weather.gov/zones/forecast/COZ068\"\n                ],\n                \"references\": [\n                    {\n                        \"@id\": \"https://api.weather.gov/alerts/urn:oid:2.49.0.1.840.0.f1520a771888f2286c7e9f041b0899cca2ffbe10.003.1\",\n                        \"identifier\": \"urn:oid:2.49.0.1.840.0.f1520a771888f2286c7e9f041b0899cca2ffbe10.003.1\",\n                        \"sender\": \"w-nws.webmaster@noaa.gov\",\n                        \"sent\": \"2025-12-03T00:40:00-07:00\"\n                    },\n                    {\n                        \"@id\": \"https://api.weather.gov/alerts/urn:oid:2.49.0.1.840.0.3e97ab4a6a3c23a3a20405d82b018ef9927db31d.003.1\",\n                        \"identifier\": \"urn:oid:2.49.0.1.840.0.3e97ab4a6a3c23a3a20405d82b018ef9927db31d.003.1\",\n                        \"sender\": \"w-nws.webmaster@noaa.gov\",\n                        \"sent\": \"2025-12-03T00:46:00-07:00\"\n                    },\n                    {\n                        \"@id\": \"https://api.weather.gov/alerts/urn:oid:2.49.0.1.840.0.b7b2384d0cd65fff536137c85933eace889e9254.003.1\",\n                        \"identifier\": \"urn:oid:2.49.0.1.840.0.b7b2384d0cd65fff536137c85933eace889e9254.003.1\",\n                        \"sender\": \"w-nws.webmaster@noaa.gov\",\n                        \"sent\": \"2025-12-03T00:53:00-07:00\"\n                    },\n                    {\n                        \"@id\": \"https://api.weather.gov/alerts/urn:oid:2.49.0.1.840.0.5bb2b589973a618ffa88ed552c21d1806fce1897.002.1\",\n                        \"identifier\": \"urn:oid:2.49.0.1.840.0.5bb2b589973a618ffa88ed552c21d1806fce1897.002.1\",\n                        \"sender\": \"w-nws.webmaster@noaa.gov\",\n                        \"sent\": \"2025-12-03T02:10:00-07:00\"\n                    }\n                ],\n                \"sent\": \"2025-12-03T08:17:00-07:00\",\n                \"effective\": \"2025-12-03T08:17:00-07:00\",\n                \"onset\": \"2025-12-03T08:17:00-07:00\",\n                \"expires\": \"2025-12-03T16:30:00-07:00\",\n                \"ends\": \"2025-12-04T02:00:00-07:00\",\n                \"status\": \"Actual\",\n                \"messageType\": \"Update\",\n                \"category\": \"Met\",\n                \"severity\": \"Moderate\",\n                \"certainty\": \"Likely\",\n                \"urgency\": \"Expected\",\n                \"event\": \"Winter Weather Advisory\",\n                \"sender\": \"w-nws.webmaster@noaa.gov\",\n                \"senderName\": \"NWS Pueblo CO\",\n                \"headline\": \"Winter Weather Advisory issued December 3 at 8:17AM MST until December 4 at 2:00AM MST by NWS Pueblo CO\",\n                \"description\": \"* WHAT...Snow. Additional snow accumulations between 4 and 12 inches.\\n\\n* WHERE...La Garita Mountains Above 10000 Feet, Eastern San Juan\\nMountains Above 10000 Feet, and Upper Rio Grande Valley/Eastern\\nSan Juan Mountains Below 10000 Feet.\\n\\n* WHEN...Until 2 AM MST Thursday.\\n\\n* IMPACTS...Travel could be very difficult. The hazardous conditions\\ncould impact the Wednesday evening commute.\",\n                \"instruction\": \"Slow down and use caution while traveling. The latest road\\nconditions for the state you are calling from can be obtained by\\ncalling 5 1 1.\",\n                \"response\": \"Execute\",\n                \"parameters\": {\n                    \"AWIPSidentifier\": [\n                        \"WSWPUB\"\n                    ],\n                    \"WMOidentifier\": [\n                        \"WWUS45 KPUB 031517\"\n                    ],\n                    \"NWSheadline\": [\n                        \"WINTER WEATHER ADVISORY REMAINS IN EFFECT UNTIL 2 AM MST THURSDAY\"\n                    ],\n                    \"BLOCKCHANNEL\": [\n                        \"EAS\",\n                        \"NWEM\",\n                        \"CMAS\"\n                    ],\n                    \"VTEC\": [\n                        \"/O.CON.KPUB.WW.Y.0026.000000T0000Z-251204T0900Z/\"\n                    ],\n                    \"eventEndingTime\": [\n                        \"2025-12-04T02:00:00-07:00\"\n                    ],\n                    \"expiredReferences\": [\n                        \"w-nws.webmaster@noaa.gov,urn:oid:2.49.0.1.840.0.1683fac8dbbcced155b8c3ee102b504a61d03b48.002.1,2025-12-02T21:22:00-07:00 w-nws.webmaster@noaa.gov,urn:oid:2.49.0.1.840.0.3af7c19979dcb0fd957b60f169e1bc971c265b37.002.1,2025-12-02T14:07:00-07:00\"\n                    ]\n                },\n                \"scope\": \"Public\",\n                \"code\": \"IPAWSv1.0\",\n                \"language\": \"en-US\",\n                \"web\": \"http://www.weather.gov\",\n                \"eventCode\": {\n                    \"SAME\": [\n                        \"NWS\"\n                    ],\n                    \"NationalWeatherService\": [\n                        \"WWY\"\n                    ]\n                }\n            }\n        },\n        {\n            \"id\": \"https://api.weather.gov/alerts/urn:oid:2.49.0.1.840.0.296069c17a90f6e5215450afb7029362483104e1.004.1\",\n            \"type\": \"Feature\",\n            \"geometry\": null,\n            \"properties\": {\n                \"@id\": \"https://api.weather.gov/alerts/urn:oid:2.49.0.1.840.0.296069c17a90f6e5215450afb7029362483104e1.004.1\",\n                \"@type\": \"wx:Alert\",\n                \"id\": \"urn:oid:2.49.0.1.840.0.296069c17a90f6e5215450afb7029362483104e1.004.1\",\n                \"areaDesc\": \"Central Chaffee County Below 9000 Ft; Western/Central Fremont County Below 8500 Ft; Canon City Vicinity/Eastern Fremont County; Colorado Springs Vicinity/Southern El Paso County/Rampart Range Below 7400 Ft; Pueblo Vicinity/Pueblo County Below 6300 Feet\",\n                \"geocode\": {\n                    \"SAME\": [\n                        \"008015\",\n                        \"
